vi "Read Adapt.vi"(8 "error in (no error)":errorcluster, 11 "Parameters in":refnum<class "Parameters.lvclass">) -> (0 "error out":errorcluster, 2 "Adapt":T1, 3 "Parameters out":refnum<class "Parameters.lvclass">)   [LabVIEW 2020, in "Parameters.lvclass"]
uses:
  Parameters.lvclass
  Typedefs/Tosca-Adapt.ctl
  Typedefs/Tosca-Adaptive Track.ctl
  Typedefs/Tosca-Simple Variable.ctl
  Adaptation VIs/Tosca-Adapt Threshold Metric.ctl
  Parameters.lvclass/Parameters.ctl
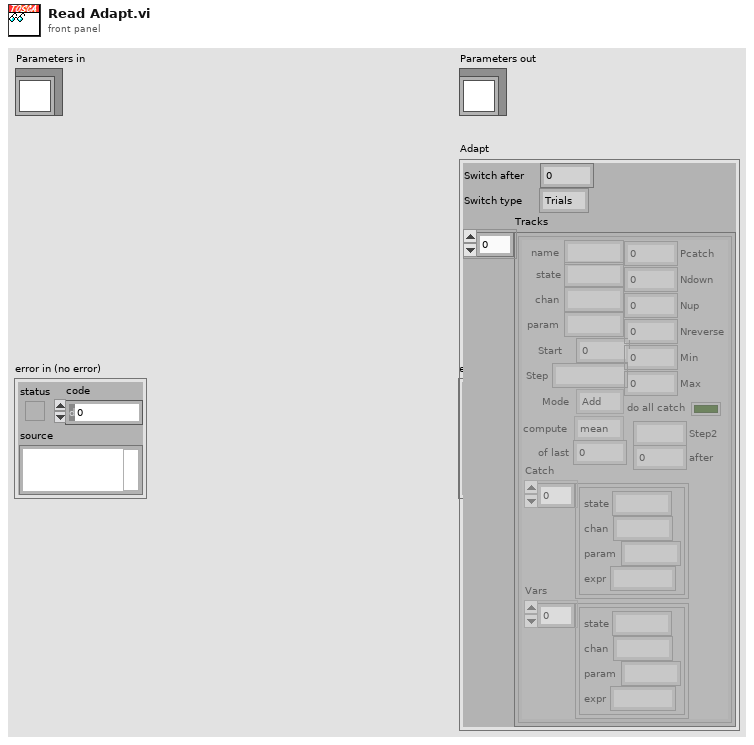
[diagram p1: front panel]
types:
  T1 = typedef "Tosca-Adapt.ctl" = cluster{"Switch after":i32, "Switch type":enum16{"Trials", "Reversals"}, "Tracks":T2[]}
  T2 = typedef "Tosca-Adaptive Track.ctl" = cluster{"state":string, "chan":string, "param":string, "Start":dbl, "Step":string, "Mode":enum16{"Add", "Multiply"}, "Pcatch":dbl, "Ndown":i32, "Nup":i32, "Nreverse":i32, "Min":dbl, "Max":dbl, "Catch":T3[], "do all catch":bool, "name":string, "Vars":T3[], "compute":T4, "of last":i32, "Step2":string, "after":i32}
  T3 = typedef "Tosca-Simple Variable.ctl" = cluster{"state":string, "chan":string, "param":string, "expr":string}
  T4 = typedef "Tosca-Adapt Threshold Metric.ctl" = enum16{"mean", "median"}
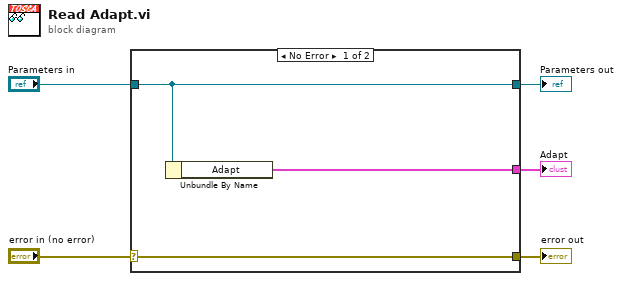
[diagram p0: block diagram]
diagram:
  n1 = case shown="No Error" "error in (no error)" {
    selector: "error in (no error)" -> [w8 w9]
    tunnel: [w8 w9] -> w4
    tunnel: [w7 w10] -> w2
    tunnel: "Parameters in" -> [w7 w10]
    tunnel: [w6 _] -> w1
    frame No Error {
      n2 = Unbundle By Name(w7) -> ("Adapt"=w6:T1)
    }
    frame Error {
    }
  }
  "error out" <- w4
  "Parameters out" <- w2
  "Adapt" <- w1
